vi "Discard Sensor Object.vi"(8 "error in (no error)":errorcluster caption="错误输入（无错误）", 11 "sensorHandle":i32) -> (0 "error out":errorcluster caption="错误输出", 3 "function return":i32)   [LabVIEW 2018]
doc: "extern int __stdcall APSxDiscardSensorObject (int sensorHandle);"
uses:
  APSx.dll/APSx.dll
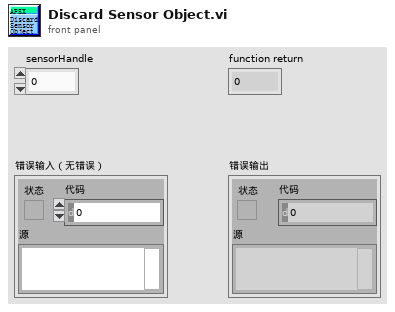
[diagram p1: front panel]
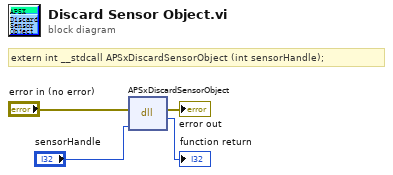
[diagram p0: block diagram]
diagram:
  # "extern int __stdcall APSxDiscardSensorObject (int sensorHandle);"
  n1 = dll-call lib="PTH2[abs D项目Feng恒隆项目Labview传感器对中台SourcesAPSx.dllAPSx.*" fn="APSxDiscardSensorObject"(error in="error in (no error)", "sensorHandle"="sensorHandle") -> (error out=→"error out":errorcluster, →"function return":i32)  [unwired: 3 in, 1 out]
